vi "Build Roles.vi"(8 "error in (no error)":errorcluster, 10 "Roles":map{string, T1}(c390), 11 "Role Manager in":refnum<class "Role Manager.lvclass">) -> (0 "error out":errorcluster, 3 "Role Manager out":refnum<class "Role Manager.lvclass">)   [LabVIEW 2020, in "Volatus.lvlib" / "Role Manager.lvclass"]
uses:
  Role Manager.lvclass
  Role.ctl
  Role Manager.lvclass/Role Manager.ctl
  Role Info.ctl
  Volatus.lvlib
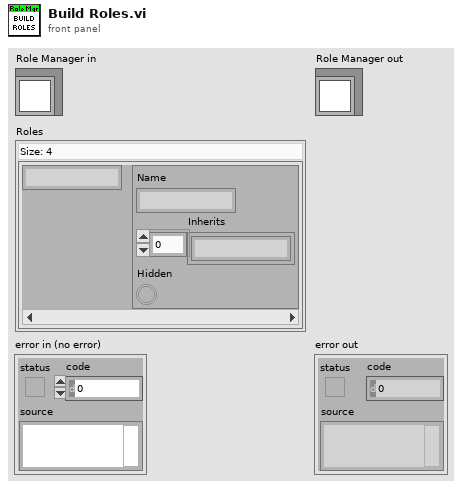
[diagram p1: front panel]
types:
  T1 = typedef "Volatus.lvlib/Role.ctl" = cluster{"Name":string, "Inherits":string[], "Hidden":bool}
  T2 = typedef "Volatus.lvlib/Role Manager.lvclass/Role Info.ctl" = cluster{"Name":string, "Hidden":bool, "Effective Roles":set{string}}
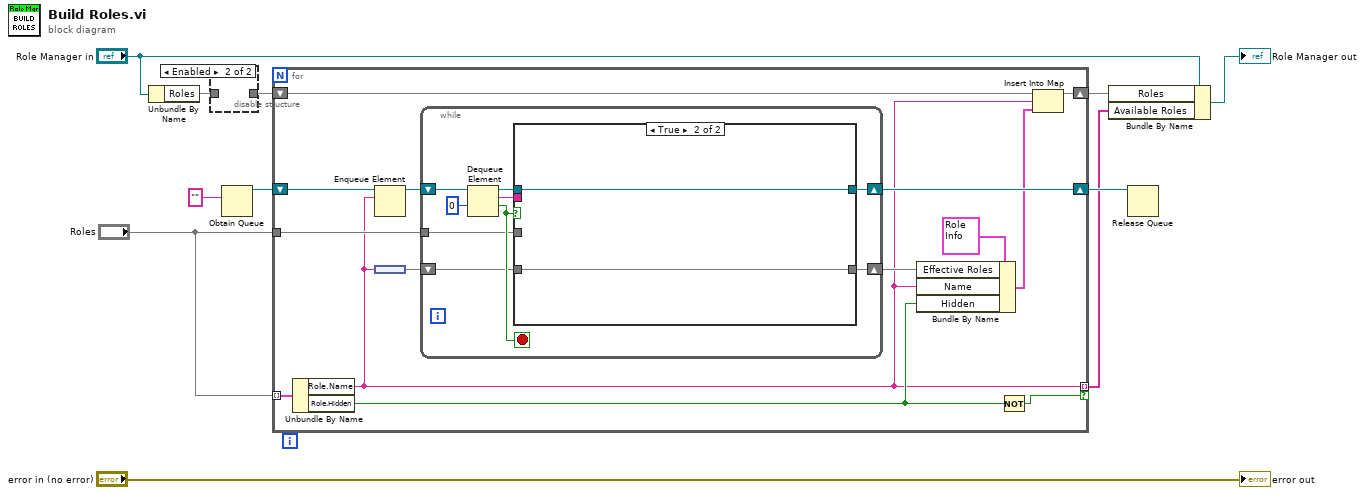
[diagram p0: block diagram]
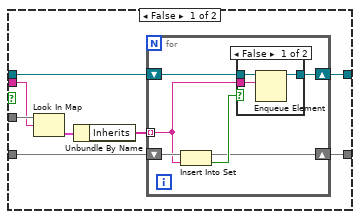
[diagram p2: hidden frame]
diagram:
  n1 = Unbundle By Name("Role Manager in") -> ("Roles"=w9:map{string, T2})
  n2 = disable-structure shown="Enabled" {
    disable-tunnel: w9 -> [w12 _]
    disable-tunnel: [w12 _] -> w8
    frame Disabled {
    }
    frame Enabled {
    }
  }
  n3 = Obtain Queue(element data type="") -> (queue out=w5:refnum<queue>)  [unwired: 4 in, 2 out]
  n4 = for {
    shift-right: [w15] -> w2
    shift-left: w8 -> [w16]
    tunnel: "Roles" -> [w26] mode=indexing
    tunnel: "Roles" -> [w22]
    tunnel: [w14] -> w1 mode=indexing if=w25
    shift-right: [w20] -> w4
    shift-left: w5 -> [w24]
    n5 = Unbundle By Name(w26) -> ("Role.Name"=w14:string, "Role.Hidden"=w17:bool)
    n6 = Enqueue Element(queue=w24, element=w14) -> (queue out=w23:refnum<queue>)  [unwired: 2 in, 2 out]
    n7 = node(w14) -> (w21:set{string})
    n8 = while {
      shift-right: [w30] -> w20
      shift-left: w23 -> [w35]
      tunnel: w22 -> [w27]
      shift-right: [w28] -> w18
      shift-left: w21 -> [w29]
      stop <- w33 stop-if-true
      n9 = Dequeue Element(queue=w35, timeout in ms (-1)=0) -> (queue out=w31:refnum<queue>, element=w32:string, timed out?=w33:bool)  [unwired: 1 in, 1 out]
      n10 = case shown="True" w33 {
        tunnel: w32 -> [w42 _]
        tunnel: w31 -> [w39 w55]
        tunnel: [w36 w55] -> w30
        tunnel: w29 -> [w38 w54]
        tunnel: [w37 w54] -> w28
        tunnel: w27 -> [w43 _]
        frame False {
          n11 = Look In Map(map=w43, key=w42) -> (value=w41:T1)  [unwired: 1 in, 1 out]
          n12 = Unbundle By Name(w41) -> ("Inherits"=w40:string[])
          n13 = for {
            tunnel: w40 -> [w46] mode=indexing
            shift-right: [w45] -> w36
            shift-left: w39 -> [w47]
            shift-right: [w44] -> w37
            shift-left: w38 -> [w49]
            n14 = Insert Into Set(10:w46, 11:w49) -> (2:w48:bool, 3:w44:set{string})
            n15 = case shown="False" w48 {
              tunnel: w47 -> [w52 w53]
              tunnel: w46 -> [w51 _]
              tunnel: [w50 w53] -> w45
              frame False {
                n16 = Enqueue Element(queue=w52, element=w51) -> (queue out=w50:refnum<queue>)  [unwired: 2 in, 2 out]
              }
              frame True {
              }
            }
          }
        }
        frame True {
        }
      }
    }
    n17 = Bundle By Name(cluster=T2 {"Name"="", "Hidden"=FALSE, "Effective Roles"={}} ("Role Info"), "Effective Roles"=w18, "Name"=w14, "Hidden"=w17) -> (w13:T2)
    n18 = Not(x=w17) -> (.not. x?=w25:bool)
    n19 = Insert Into Map(map in=w16, key=w14, value=w13) -> (map out=w15:map{string, T2})  [unwired: 2 out]
  }
  n20 = Bundle By Name(cluster="Role Manager in", "Roles"=w2, "Available Roles"=w1) -> (→"Role Manager out":refnum<class "Role Manager.lvclass">)
  n21 = Release Queue(queue=w4) -> ()  [unwired: 2 in, 3 out]
  "error out" <- "error in (no error)"
